vi "FPGA_DIOOpen.vi"(8 "error in (no error)":errorcluster) -> (0 "error out":errorcluster, 3 "DIODeviceRef":T1)   [LabVIEW 2017]
uses:
  <vilib>/Rock Robotics/SystemInterfaces/DIO/FPGA_DIODevRef.ctl
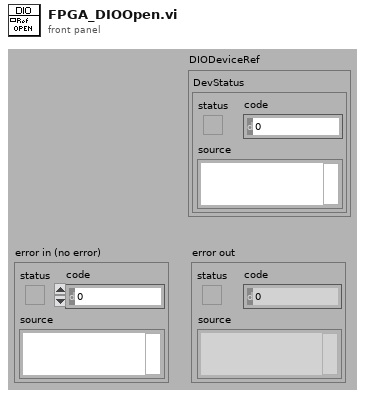
[diagram p1: front panel]
types:
  T1 = typedef "FPGA_DIODevRef.ctl" = cluster{"DevStatus":errorcluster}
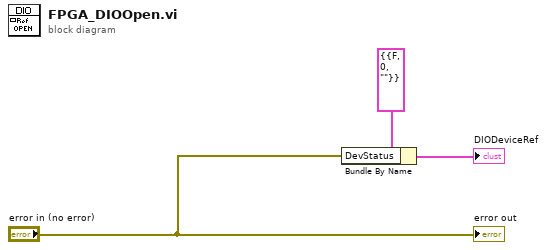
[diagram p0: block diagram]
diagram:
  n1 = Bundle By Name(cluster=T1 {"DevStatus"={"status"=FALSE, "code"=0, "source"=""}} ("DIODeviceRef"), "DevStatus"="error in (no error)") -> (→"DIODeviceRef":T1)
  "error out" <- "error in (no error)"
